vi "Simu_sinus_Pid_For.vi"() -> ()   [LabVIEW 2026]
uses:
  <vilib>/Analysis/1siggen.llb/Ramp Pattern by Samples.vi
  <vilib>/addons/control/pid/pid.llb/PID (DBL).vi
  <vilib>/addons/control/pid/NI_PID_pid.lvlib
  <vilib>/Analysis/NI_AALBase.lvlib
panel:
  out "Tableau":dbl[](array[numeric])
  out "Tension":dbl[](array[numeric]) caption="Motif de rampe"
  out "VP out":dbl[](array[numeric])
  out "PID out":dbl[](array[numeric])
  out "Ramp Pattern":dbl[](array[numeric]) caption="Motif de rampe"
  out "output":dbl caption="sortie" format="%.2f"
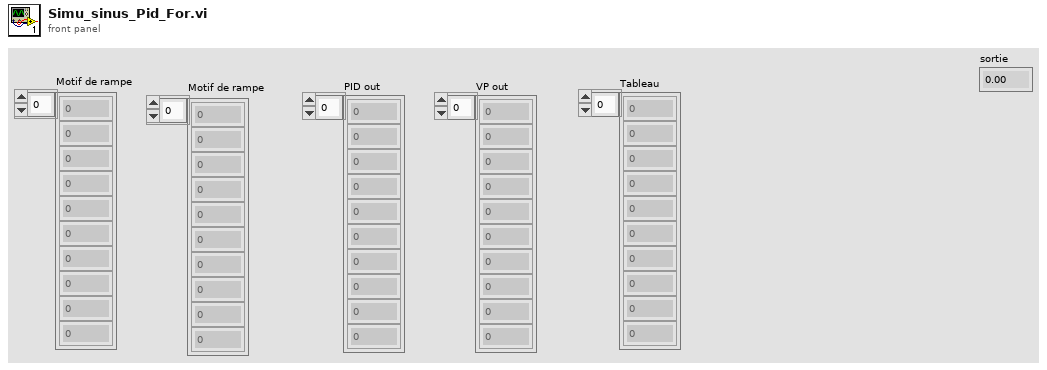
[diagram p1: front panel]
types:
  T1 = cluster{"proportional gain (Kc)":dbl, "integral time (Ti, min)":dbl, "derivative time (Td, min)":dbl}
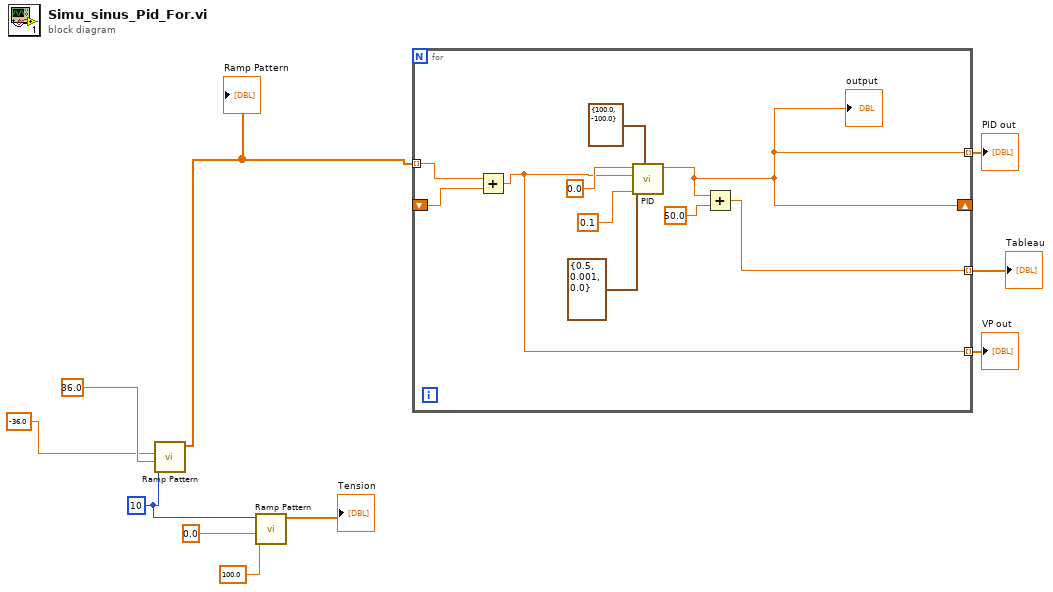
[diagram p0: block diagram]
diagram:
  w7 = 10 ("samples")
  n1 = call-poly <vilib>:"Ramp Pattern.vi"("start"=36.0 ("end"), "end"=-36.0 ("start"), "samples"=w7) -> ("Ramp Pattern"=w10:dbl[])  [unwired: 7 in, 1 out]
  "Ramp Pattern" <- w10
  n2 = call-poly <vilib>:"Ramp Pattern.vi"("start"=0.0, "end"=100.0, "samples"=w7) -> ("Ramp Pattern"=→"Tension":dbl[])  [unwired: 7 in, 1 out]
  n3 = for {
    tunnel: w10 -> [w16] mode=indexing
    shift-right: [w11] -> _
    shift-left: _ -> [w15]
    tunnel: [w11] -> w9 mode=indexing
    tunnel: [w14] -> w8 mode=indexing
    tunnel: [w12] -> w1 mode=indexing
    n4 = Add(x=w16, y=w15) -> (x+y=w14:dbl)
    n5 = call-poly <vilib>:"PID.vi"("output range"=cluster{"output high":dbl, "output low":dbl} {"output high"=100.0, "output low"=-100.0}, "dt (s)"=0.1, "PID gains"=T1 {"proportional gain (Kc)"=0.5, "integral time (Ti, min)"=0.001, "derivative time (Td, min)"=0.0}, "process variable"=w14, "setpoint"=0.0) -> ("output"=w11:dbl)  [unwired: 5 in, 1 out]
    "output" <- w11
    n6 = Add(x=w11, y=50.0) -> (x+y=w12:dbl)
  }
  "PID out" <- w9
  "VP out" <- w8
  "Tableau" <- w1
